vi "ReadSpreadsheetFile(DBL).vi"(6 "Format(%.3f)":string="%.3f", 7 "Delimiter(\\t)":string="\t", 8 "ErrorIn":errorcluster, 11 "FilePathIn":path) -> (0 "ErrorOut":errorcluster, 1 "FirstRow":dbl[](array[numeric]), 2 "DataOut":dbl[][](array[numeric]), 3 "FilePathOut":path)   [LabVIEW 2018]
doc: "Reads the contents of a string and tab delimeted text file and converts the data to a 2D, double-precision array of numbers, strings, or integers.\n\nCopyright © 2011 Epimedia, Inc. All Rights Reserved.\n\nThe Epimedia Application Library is Copyright © 2009-2011 Epimedia, Inc. \nAll Rights Reserved. Used under license."
panel:
  # "Copyright © 2011 Epimedia, Inc. All Rights Reserved.\n\nThe Epimedia Application Library is Copyright © 2009-2011 Epimedia, Inc. \nAll Rights Reserved. Used under license."
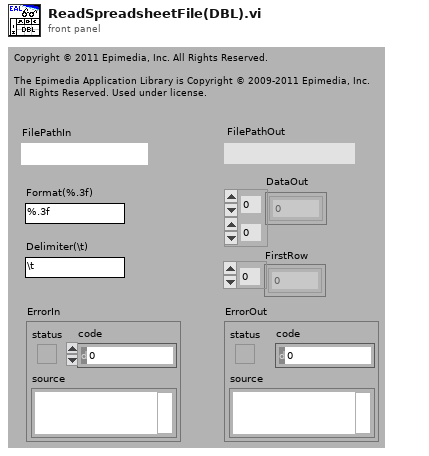
[diagram p1: front panel]
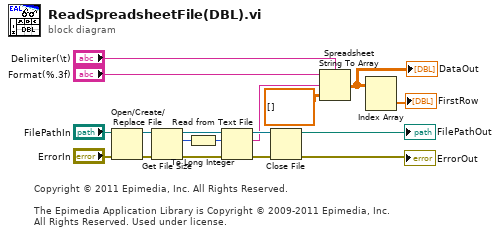
[diagram p0: block diagram]
diagram:
  # "Copyright © 2011 Epimedia, Inc. All Rights Reserved.\n\nThe Epimedia Application Library is Copyright © 2009-2011 Epimedia, Inc. \nAll Rights Reserved. Used under license."
  n1 = Open/Create/Replace File(file path (use dialog)="FilePathIn", error in="ErrorIn") -> (refnum out=w7:refnum<file>, error out=w8:errorcluster)  [unwired: 4 in, 1 out]
  n2 = Get File Size(file=w7, error in=w8) -> (refnum out=w6:refnum<file>, size (in bytes)=w4:i64, 0:w5:errorcluster)
  n3 = To Long Integer(number=w4) -> (32bit integer=w3:i32)
  n4 = Read from Text File(file (use dialog)=w6, count=w3, error in=w5) -> (refnum out=w13:refnum<file>, text=w9:string, error out=w14:errorcluster)  [unwired: 1 in, 1 out]
  n5 = Close File(refnum=w13, error in=w14) -> (path=→"FilePathOut":path, error out=→"ErrorOut":errorcluster)
  n6 = Spreadsheet String To Array(delimiter (Tab)="Delimiter(\\t)", format string="Format(%.3f)", spreadsheet string=w9, array type (2D Dbl)=dbl[][] [] ("type (empty)")) -> (array=w2:dbl[][])
  "DataOut" <- w2
  n7 = Index Array(array=w2) -> (element=→"FirstRow":dbl[])  [unwired: 2 in]
